vi "Upload Firmware.vi"(5 "Progress Bar":refnum<vi>, 6 "AVRDUDE Timeout (15000)":u32=15000, 7 "COM Port":refnum<visa-resource-name>="COM5", 8 "Error In":errorcluster, 9 "Firmware Version":u16(ring) items=["LINX -  Serial / USB", "LINX -  Serial / USB [Debug] "], 10 "Device ID":u16=1, 11 "Device Family":T1=enum."Digilent") -> (0 "Error Out":errorcluster={"status"=TRUE, "code"=-1073807346, "source"="VISA Open in LVH-LINX.lvlib:Upload Firmware.vi"}, 2 "Success?":bool)   [LabVIEW 2013, in "LVH-LINX.lvlib"]
uses:
  <vilib>/LabVIEW Hacker/LINX/LVH-LINX.lvlib
  <vilib>/LabVIEW Hacker/LINX/Private/Type Defs/Devices - Arduino.ctl
  <vilib>/LabVIEW Hacker/LINX/Private/Type Defs/Devices - Digilent.ctl
  <vilib>/LabVIEW Hacker/LINX/Private/Device/Device.lvlib
  <vilib>/LabVIEW Hacker/LINX/Private/Type Defs/Device Family.ctl
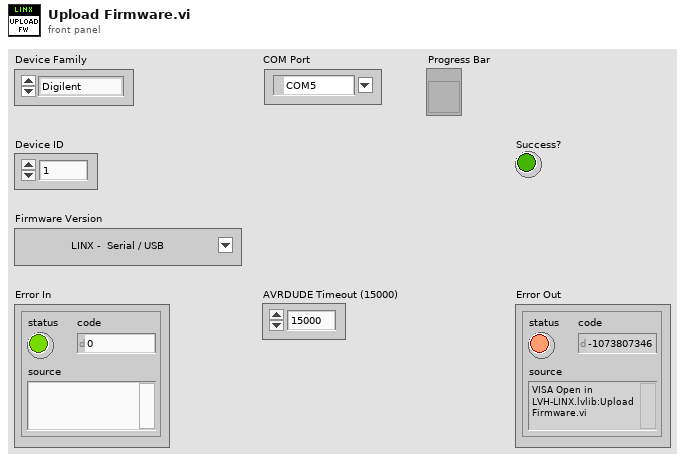
[diagram p1: front panel]
types:
  T1 = typedef "LVH-LINX.lvlib/Device Family.ctl" = enum8{"National Instruments", "Digilent", "Arduino"}
  T2 = typedef "LVH-LINX.lvlib/Generic Device.ctl" = cluster{"DI Channels":u8[], "DO Channels":u8[], "AI":u8[], "AO":u8[], "PWM":u8[], "QE":u8[], "UART":u8[], "I2C 2":u8[], "SPI":u8[], "CAN":u8[], "AI Ref (V)":dbl, "Firmware Program Interfaces":enum16{"N/A", "Serial / USB", "USB", "TCP"}[], "Firmware Versions":T3[], "Name":string, "AO Resolution (Bits)":u8, "AO Ref (V)":dbl}
  T3 = typedef "LVH-LINX.lvlib/Firmware Version.ctl" = cluster{"Name":string, "Relative Path":string, "Firmware Interface":T4}
  T4 = typedef "LVH-LINX.lvlib/Firmware Interface.ctl" = enum32{"Serial ", "Ethernet", "WIFI"}
  T5 = typedef "LVH-LINX.lvlib/Devices - Digilent.ctl" = enum16{"chipKIT Uno32", "chipKIT uC32", "chipKIT Max32", "chipKIT WF32"}
  T6 = typedef "LVH-LINX.lvlib/Devices - Arduino.ctl" = enum16{"Uno", "Mega 2560", "Leonardo", "Due", "Yun", "Nano", "Pro Mini", "Pro", "Fio", "Mega1280"}
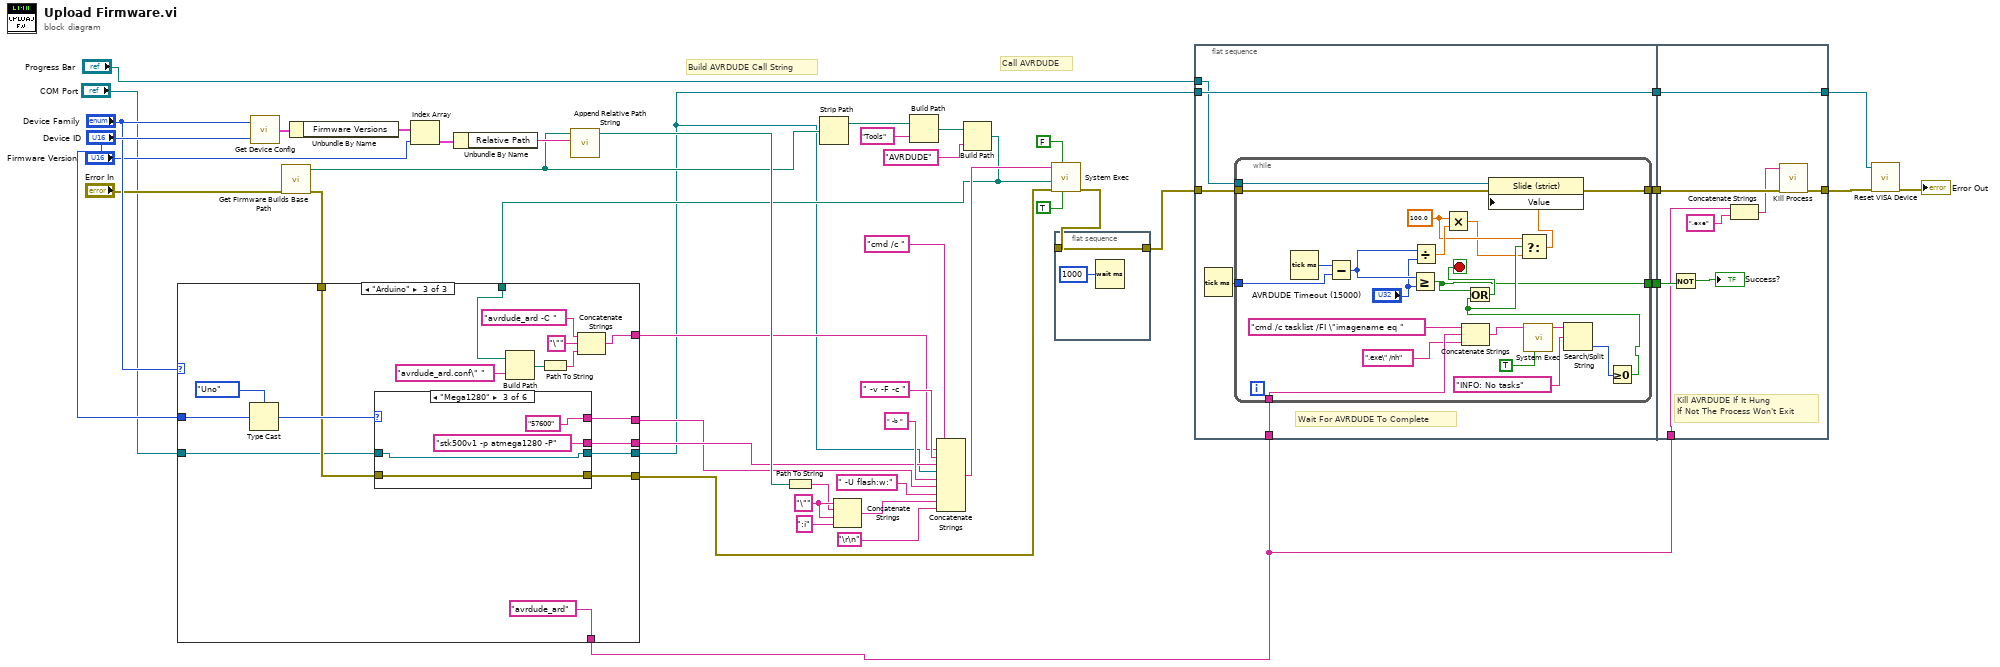
[diagram p0: block diagram]
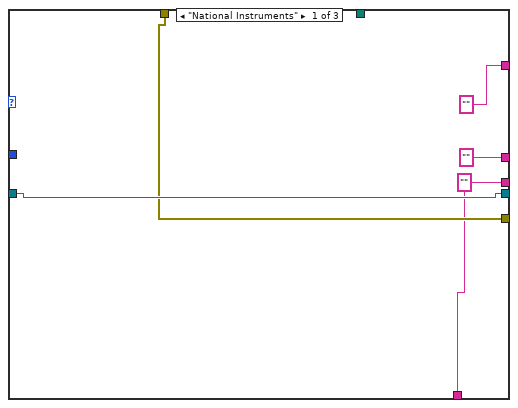
[diagram p2: hidden frame]
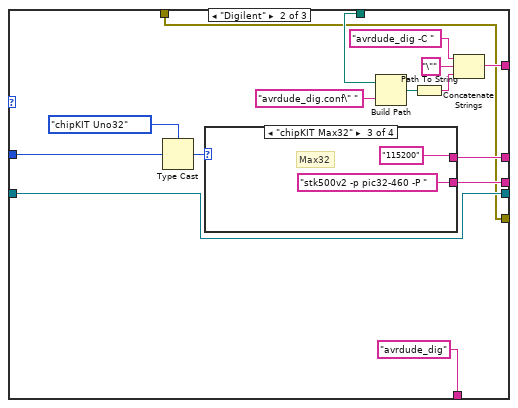
[diagram p3: hidden frame]
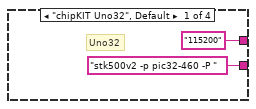
[diagram p4: hidden frame]
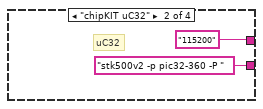
[diagram p5: hidden frame]
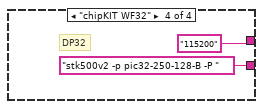
[diagram p6: hidden frame]
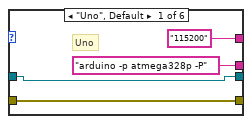
[diagram p7: hidden frame]
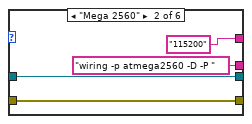
[diagram p8: hidden frame]
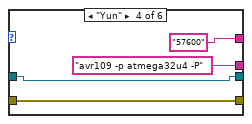
[diagram p9: hidden frame]
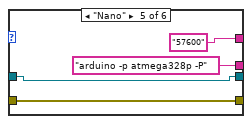
[diagram p10: hidden frame]
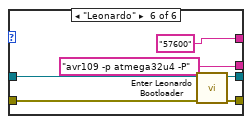
[diagram p11: hidden frame]
diagram:
  w41 = "\"" ("string")
  # "Call AVRDUDE"
  # "Build AVRDUDE Call String"
  n1 = call <vilib>:"Get Device Config.vi"("Device ID"="Device ID", "Device Family"="Device Family") -> ("Device Config"=w24:T2)
  n2 = call <vilib>:"Get Firmware Builds Base Path.vi"("Error In"="Error In") -> ("Error Out"=w8:errorcluster, "Firmware Builds Base Path"=w35:path)  [unwired: 9 in]
  n3 = Unbundle By Name(w24) -> ("Firmware Versions"=w25:T3[])
  n4 = Index Array(array=w25, index="Firmware Version") -> (element=w36:T3)
  n5 = Unbundle By Name(w36) -> ("Relative Path"=w37:string)
  n6 = call <vilib>:"Append Relative Path String.vi"("Relative Path"=w37, "Base Path"=w35) -> ("Absolute Path"=w39:path)  [unwired: 8 in, 1 out]
  n7 = Path To String(path=w39) -> (string=w40:string)
  n8 = Strip Path(path=w35) -> (stripped path=w28:path)  [unwired: 1 out]
  n9 = Concatenate Strings(w41, w40, w41, ":i" ("string")) -> (w15:string)
  n10 = Build Path(base path=w28, name or relative path="Tools") -> (appended path=w30:path)
  n11 = Build Path(base path=w30, name or relative path="AVRDUDE") -> (appended path=w9:path)
  n12 = case shown="\"Arduino\"" "Device Family" {
    tunnel: [w45 w64 w86] -> w32
    tunnel: "Device ID" -> [_ w62 w87]
    tunnel: ["" ("string") w60 w85] -> w13
    tunnel: ["" ("string") w56 w80] -> w11
    tunnel: w9 -> [_ w59 w79]
    tunnel: w8 -> [w47 w52 w78]
    tunnel: [w47 w52 w77] -> w7
    tunnel: "COM Port" -> [w48 w53 w76]
    tunnel: [w48 w53 w75] -> w5
    tunnel: [w45 "avrdude_dig" ("string") "avrdude_ard" ("string")] -> w1
    frame "National Instruments" {
      w45 = "" ("string")
    }
    frame "Digilent" {
      n13 = Type Cast(type=Devices_-_Digilent."chipKIT Uno32" ("Digilent Device"), x=w62) -> (*(type *) &x=w63:T5)
      n14 = case shown="\"chipKIT Max32\"" w63 {
        tunnel: ["stk500v2 -p pic32-460 -P " ("string") "stk500v2 -p pic32-360 -P " ("string") "stk500v2 -p pic32-460 -P " ("string") "stk500v2 -p pic32-250-128-B -P " ("string")] -> w64
        tunnel: ["115200" ("string") "115200" ("string") "115200" ("string") "115200" ("string")] -> w60
        frame "chipKIT Uno32", Default {
          # "Uno32"
        }
        frame "chipKIT uC32" {
          # "uC32"
        }
        frame "chipKIT Max32" {
          # "Max32"
        }
        frame "chipKIT WF32" {
          # "DP32"
        }
      }
      n15 = Build Path(base path=w59, name or relative path="avrdude_dig.conf\" ") -> (appended path=w57:path)
      n16 = Path To String(path=w57) -> (string=w54:string)
      n17 = Concatenate Strings("avrdude_dig -C " ("string"), "\"" ("string"), w54) -> (w56:string)
    }
    frame "Arduino" {
      n18 = Type Cast(type=Devices_-_Arduino."Uno" ("Arduino Device"), x=w87) -> (*(type *) &x=w88:T6)
      n19 = case shown="\"Mega1280\"" w88 {
        tunnel: ["arduino -p atmega328p -P" "wiring -p atmega2560 -D -P " "stk500v1 -p atmega1280 -P" "avr109 -p atmega32u4 -P" "arduino -p atmega328p -P" "avr109 -p atmega32u4 -P"] -> w86
        tunnel: ["115200" ("string") "115200" ("string") "57600" ("string") "57600" ("string") "57600" ("string") "57600" ("string")] -> w85
        tunnel: w78 -> [w90 w94 w98 w102 w106 w113]
        tunnel: [w90 w94 w98 w102 w106 w112] -> w77
        tunnel: w76 -> [w91 w95 w99 w103 w107 w111]
        tunnel: [w91 w95 w99 w103 w107 w110] -> w75
        frame "Uno", Default {
          # "Uno"
        }
        frame "Mega 2560" {
        }
        frame "Mega1280" {
        }
        frame "Yun" {
        }
        frame "Nano" {
        }
        frame "Leonardo" {
          n20 = call <vilib>:"Enter Leonardo Bootloader.vi"("Error In"=w113, "VISA resource name"=w111) -> ("Error Out"=w112:errorcluster, "VISA resource name"=w110:refnum<visa-resource-name>)  [unwired: 7 in, 1 out]
        }
      }
      n21 = Build Path(base path=w79, name or relative path="avrdude_ard.conf\" ") -> (appended path=w83:path)
      n22 = Path To String(path=w83) -> (string=w81:string)
      n23 = Concatenate Strings("avrdude_ard -C " ("string"), "\"" ("string"), w81) -> (w80:string)
    }
  }
  n24 = Concatenate Strings("cmd /c " ("string"), w11, " -v -F -c " ("string"), w32, w5, " -b " ("string"), w13, " -U flash:w:" ("string"), w15, "\r\n") -> (w23:string)
  n25 = call <vilib>:"System Exec.vi"("run minimized? (F)"=TRUE, "wait until completion? (T)"=FALSE, "error in (no error)"=w7, "working directory"=w9, "command line"=w23) -> ("error out"=w3:errorcluster)  [unwired: 3 in, 3 out]
  n26 = flat-sequence {
    tunnel: [w117] -> w2
    tunnel: w3 -> [w117]
    frame #0 {
      n27 = Wait (ms)(milliseconds to wait=u32 1000) -> ()  [unwired: 1 out]
    }
  }
  n28 = flat-sequence {
    tunnel: w2 -> [w121]
    tunnel: [w122] -> w22
    tunnel: [w123] -> w21
    tunnel: w5 -> [w123]
    tunnel: "Progress Bar" -> [w120]
    tunnel: [w119] -> w4
    tunnel: w1 -> [w118]
    tunnel: w22 -> [w154]
    tunnel: w21 -> [w152]
    tunnel: [w153] -> w19
    tunnel: [w152] -> w17
    tunnel: w4 -> [w151]
    tunnel: w1 -> [w149]
    frame #0 {
      # "Wait For AVRDUDE To Complete"
      n29 = Tick Count (ms)() -> (millisecond timer value=w124:u32)
      n30 = while {
        tunnel: w124 -> [w145]
        tunnel: [w144] -> w122
        tunnel: w121 -> [w143]
        tunnel: w120 -> [w142]
        tunnel: [w129] -> w119
        tunnel: w118 -> [w126]
        stop <- w135 stop-if-true
        w132 = 100.0 ("x")
        n31 = Tick Count (ms)() -> (millisecond timer value=w146:u32)
        n32 = Subtract(x=w146, y=w145) -> (x-y=w141:u32)
        n33 = Greater Or Equal?(x=w141, y="AVRDUDE Timeout (15000)") -> (x >= y?=w129:bool)
        n34 = Divide(x=w141, y="AVRDUDE Timeout (15000)") -> (x/y=w139:dbl)
        n35 = Multiply(x=w132, y=w139) -> (x*y=w131:dbl)
        n36 = Concatenate Strings("cmd /c tasklist /FI \"imagename eq " ("command line"), w126, ".exe\" /nh" ("string")) -> (w127:string)
        n37 = call <vilib>:"System Exec.vi"("run minimized? (F)"=TRUE, "command line"=w127) -> ("standard output"=w137:string)  [unwired: 6 in, 3 out]
        n38 = Search/Split String(string=w137, search string/char (-)="INFO: No tasks") -> (offset of match=w134:i32)  [unwired: 1 in, 2 out]
        n39 = Greater Or Equal To 0?(x=w134) -> (x >= 0?=w133:bool)
        n40 = Or(x=w129, y=w133) -> (x .or. y?=w135:bool)
        n41 = Select(t=w132, s=w133, f=w131) -> (s? t:f=w130:dbl)
        n42 = property class="Slide (strict)"(reference=w142, error in=w143, "Value"=w130) -> (error out=w144:errorcluster)  [unwired: 1 out]
      }
    }
    frame #1 {
      # "Kill AVRDUDE If It Hung\nIf Not The Process Won't Exit"
      n43 = Not(x=w151) -> (.not. x?=→"Success?":bool)
      n44 = Concatenate Strings(w149, ".exe" ("string")) -> (w147:string)
      n45 = call <vilib>:"Kill Process.vi"("Error In"=w154, "Process Name"=w147) -> ("Error Out"=w153:errorcluster)  [unwired: 9 in]
    }
  }
  n46 = call <vilib>:"Reset VISA Device.vi"("Error In"=w19, "VISA resource name"=w17) -> ("Error Out"=→"Error Out":errorcluster)  [unwired: 9 in]
